vi "HFRR ADV v13.vi"() -> ()   [LabVIEW 2025] (continued)
                      n3139 = Fract/Exp String To Number(string=w4398) -> (number=→"Temperature before test 2":dbl)  [unwired: 3 in, 1 out]
                    }
                    frame 8 {
                      n3140 = Fract/Exp String To Number(string=w4400) -> (number=→"Humidity after test 2":dbl)  [unwired: 3 in, 1 out]
                    }
                    frame 9 {
                      n3141 = Fract/Exp String To Number(string=w4402) -> (number=→"Temperature after test 2":dbl)  [unwired: 3 in, 1 out]
                    }
                    frame 10 {
                      n3142 = Fract/Exp String To Number(string=w4404) -> (number=→"MWSD 2":dbl)  [unwired: 3 in, 1 out]
                    }
                    frame 11 {
                      n3143 = Fract/Exp String To Number(string=w4406) -> (number=→"AVP 2":dbl)  [unwired: 3 in, 1 out]
                    }
                    frame 12 {
                      n3144 = Fract/Exp String To Number(string=w4408) -> (number=→"HCF 2":dbl)  [unwired: 3 in, 1 out]
                    }
                    frame 13 {
                      n3145 = Fract/Exp String To Number(string=w4410) -> (number=→"WS1.4 2":dbl)  [unwired: 3 in, 1 out]
                    }
                    frame 14, Default {
                    }
                  }
                }
              }
              frame #2 {
              }
            }
            n3146 = local write "OK Button 16"(FALSE ("OK Button 13")) -> ()
          }
        }
        n3147 = Index Array(array=w4054, index="Select Printer 3") -> (element=w4056:string)
        "Selected Printer" <- w4056
        n3148 = case shown="True" w4051 {
          frame False {
          }
          frame True {
            n3149 = flat-sequence {
              frame #0 {
              }
              frame #1 {
                n3150 = Wait (ms)(milliseconds to wait=u32 100) -> ()  [unwired: 1 out]
              }
              frame #2 {
                n3151 = local write "OK Button 16"(FALSE ("Print 3")) -> ()
              }
            }
          }
        }
        n3152 = case shown="True" "Print" {
          tunnel: w4056 -> [_ w4348]
          frame False {
          }
          frame True {
            (unwired) i16 6 ("width (-)")
            (unwired) "TESTED BY : "
            (unwired) "TESTED DATE :"
            (unwired) "SAMPLE ID : "
            (unwired) "SAMPLE DESIGN : "
            w4306 = "\r"
            w4323 = "\r"
            # "add image"
            n3153 = local read "Sample ID"() -> (w4296:string)
            n3154 = local read "Tested by"() -> (w4299:string)
            n3155 = local read "String 34"() -> (w4286:string)
            n3156 = local read "String 45"() -> (w4266:string)
            n3157 = local read "String 35"() -> (w4281:string)
            n3158 = local read "String 37"() -> (w4279:string)
            n3159 = local read "String 32"() -> (w4301:string)
            n3160 = local read "String 36"() -> (w4276:string)
            n3161 = local read "String 31"() -> (w4300:string)
            n3162 = local read "Test Date"() -> (w4297:string)
            n3163 = local read "String 33"() -> (w4302:string)
            n3164 = local read "String 38"() -> (w4272:string)
            n3165 = local read "String 39"() -> (w4269:string)
            n3166 = local write "Print"(FALSE ("Print FF")) -> ()
            n3167 = local read "S 39"() -> (w4284:string)
            n3168 = local read "S 38"() -> (w4291:string)
            n3169 = local read "Temperature before test 2"() -> (w4322:dbl)
            n3170 = local read "Temperature after test 2"() -> (w4312:dbl)
            n3171 = local read "Humidity before test 2"() -> (w4337:dbl)
            n3172 = local read "Humidity after test 2"() -> (w4321:dbl)
            n3173 = local read "MWSD 2"() -> (w4326:dbl)
            n3174 = local read "WS1.4 2"() -> (w4304:dbl)
            n3175 = Concatenate Strings("2)" ("string"), w4286) -> (w4287:string)
            n3176 = Concatenate Strings("3)" ("string"), w4284) -> (w4285:string)
            n3177 = Concatenate Strings("1)" ("string"), w4291) -> (w4290:string)
            n3178 = Concatenate Strings("4)" ("string"), w4281) -> (w4282:string)
            n3179 = Concatenate Strings("5)" ("string"), w4279) -> (w4278:string)
            n3180 = Concatenate Strings("6)" ("string"), w4276) -> (w4275:string)
            n3181 = Concatenate Strings("7)" ("string"), w4272) -> (w4273:string)
            n3182 = Concatenate Strings("8)" ("string"), w4269) -> (w4270:string)
            n3183 = local read "HCF 2"() -> (w4308:dbl)
            n3184 = local read "AVP 2"() -> (w4325:dbl)
            n3185 = local read "s.NO"() -> (w4267:string)
            n3186 = call <vilib>:"New Report.vi"("report type"=enum16{"Standard Report", "HTML"}."Standard Report") -> ("report out"=w4346:refnum<class "NI_report.lvclass">, "error out"=w4345:errorcluster)  [unwired: 13 in]
            n3187 = local read "TITTLE"() -> (w4298:string)
            n3188 = Concatenate Strings(w4323, w4266, w4267, w4323, w4301, w4296, w4323, w4300, w4297, w4323, w4302, w4299, w4323) -> (w4316:string)
            "test by" <- w4316
            n3189 = Number To Fractional String(number=w4322, width (-)=i16 6, precision (6)=i16 2) -> (F-format string=w4311:string)  [unwired: 1 in]
            n3190 = Number To Fractional String(number=w4321, width (-)=i16 6, precision (6)=i16 2) -> (F-format string=w4324:string)  [unwired: 1 in]
            n3191 = Number To Fractional String(number=w4337, width (-)=i16 6, precision (6)=i16 2) -> (F-format string=w4342:string)  [unwired: 1 in]
            n3192 = Number To Fractional String(number=w4326, width (-)=i16 6, precision (6)=i16 2) -> (F-format string=w4328:string)  [unwired: 1 in]
            n3193 = Number To Fractional String(number=w4312, width (-)=i16 6, precision (6)=i16 2) -> (F-format string=w4313:string)  [unwired: 1 in]
            n3194 = Number To Fractional String(number=w4325, width (-)=i16 6, precision (6)=i16 2) -> (F-format string=w4327:string)  [unwired: 1 in]
            n3195 = Number To Fractional String(number=w4308, width (-)=i16 6, precision (6)=i16 2) -> (F-format string=w4307:string)  [unwired: 1 in]
            n3196 = Number To Fractional String(number=w4304, precision (6)=i16 2) -> (F-format string=w4303:string)  [unwired: 2 in]
            n3197 = call-dynamic "Set Report Header Text.vi"("report in"=w4346, "center header text"=w4298, "error in (no error)"=w4345) -> ("report out"=w4317:refnum<class "NI_report.lvclass">, "error out"=w4318:errorcluster)  [unwired: 11 in]
            n3198 = Concatenate Strings(w4306, w4290, w4342, w4306, w4287, w4311, w4306, w4285, w4324, w4306, w4282, w4313, w4306, w4278, w4328, w4306, w4275, w4327, w4306, w4273, w4307, w4306, w4270, w4303) -> (w4294:string)
            "export 2" <- w4294
            n3199 = call-poly <vilib>:"Append Report Text.vi"("report in"=w4317, "text"=w4316, "error in (no error)"=w4318) -> ("report out"=w4320:refnum<class "NI_report.lvclass">, "error out"=w4319:errorcluster)  [unwired: 9 in, 2 out]
            n3200 = local read "test by"() -> (w4293:string)
            n3201 = local read "TITTLE"() -> (w4295:string)
            n3202 = call-poly <vilib>:"Append Report Text.vi"("report in"=w4320, "error in (no error)"=w4319) -> ("report out"=w4341:refnum<class "NI_report.lvclass">, "error out"=w4339:errorcluster)  [unwired: 10 in, 2 out]
            n3203 = Concatenate Strings(w4295, w4294, w4293) -> (→"output":string)
            n3204 = call-poly <vilib>:"Append Report Text.vi"("report in"=w4341, "text"=w4294, "error in (no error)"=w4339) -> ("report out"=w4340:refnum<class "NI_report.lvclass">, "error out"=w4338:errorcluster)  [unwired: 9 in, 2 out]
            n3205 = call-dynamic "Print Report.vi"("report in"=w4340, "printer name (default)"=w4348, "error in (no error)"=w4338) -> ("report out"=w4350:refnum<class "NI_report.lvclass">, "error out"=w4351:errorcluster)  [unwired: 11 in]
            n3206 = call-dynamic "Dispose Report.vi"("report in"=w4350, "error in (no error)"=w4351) -> ()  [unwired: 13 in, 1 out]
          }
        }
        n3207 = case shown="True" "Print 2" {
          frame False {
          }
          frame True {
            n3208 = flat-sequence {
              frame #0 {
                n3209 = local read "s.NO"() -> (→"s.NO 2":string)
                n3210 = Wait (ms)(milliseconds to wait=u32 20) -> ()  [unwired: 1 out]
                n3211 = local read "Sample ID  3"() -> (→"Sample ID  6":string)
                n3212 = local read "Sample ID  4"() -> (→"Sample ID  7":string)
                n3213 = local read "Sample ID"() -> (→"Sample ID  2":string)
                n3214 = local read "Tested by"() -> (→"Tested by 2":string)
                n3215 = local read "Test Date"() -> (→"Test Date 2":string)
                n3216 = local read "Humidity after test 3"() -> (→"Humidity after test 4":dbl)
                n3217 = local read "Ref A Test Date :"() -> (→"TITTLE 4":string)
                n3218 = local read "Temperature before test 3"() -> (w4173:dbl)
                n3219 = local read "Temperature before test 3"() -> (→"Temperature after test 5":dbl)
                n3220 = local read "Temperature after test 3"() -> (→"Temperature after test 4":dbl)
                n3221 = local read "Humidity before test 3"() -> (→"Humidity before test 4":dbl)
                n3222 = local write "Temperature before test 3"(w4173) -> ()
                n3223 = local read "image data"() -> (w4164:T14)
                n3224 = String To Path(string="C:\\LAB-IQ\\im\\Temp_resized.jpg") -> (path=w4165:path)
                "path 2" <- w4165
                n3225 = call <vilib>:"Write JPEG File.vi"("image data"=w4164, "path to JPEG file"=w4165) -> ()  [unwired: 8 in, 2 out]
                "Ref A Test Date :" <- "Ref A Test Date :"
                "Ref B Test Date :" <- "Ref B Test Date :"
                "Ref B Scar Value :" <- "Ref B Scar Value :"
                "Ref A Scar Value :" <- "Ref A Scar Value :"
              }
              frame #1 {
                (unwired) HTML_Report_Image_Alignment."MIDDLE" ("alignment (default)")
                w4201 = u16 0 items=["portrait", "landscape"] ("orientation (portrait)")
                (unwired) HTML_Report_Image_Alignment."ABSMIDDLE" ("alignment (default)")
                (unwired) "TESTED BY : "
                (unwired) "TESTED DATE :"
                (unwired) "SAMPLE ID : "
                (unwired) "SAMPLE DESIGN : "
                w4234 = "\r"
                # "add image"
                n3226 = Wait (ms)(milliseconds to wait=u32 20) -> ()  [unwired: 1 out]
                n3227 = local read "Sample ID  2"() -> (w4227:string)
                n3228 = local read "Wear Scar X"() -> (w4199:dbl)
                "Length ( microns ) 2" <- w4199
                n3229 = local read "Wear Scar Y"() -> (w4198:dbl)
                "Wear Scar Y ( microns ) :" <- w4198
                n3230 = local read "Test Date 2"() -> (w4228:string)
                n3231 = local read "Tested by 2"() -> (w4229:string)
                n3232 = local read "String 46"() -> (w4225:string)
                n3233 = local read "String 48"() -> (w4231:string)
                n3234 = local read "String 47"() -> (w4230:string)
                n3235 = local read "String 49"() -> (w4232:string)
                n3236 = local read "String 10"() -> (w4185:string)
                n3237 = local read "s.NO 2"() -> (w4226:string)
                n3238 = Add(x=w4199, y=w4198) -> (x+y=w4197:dbl)
                n3239 = call <vilib>:"New Report.vi"("report type"=enum16{"Standard Report", "HTML"}."HTML") -> ("report out"=w4205:refnum<class "NI_report.lvclass">, "error out"=w4203:errorcluster)  [unwired: 13 in]
                n3240 = Concatenate Strings(w4234, w4225, w4226, w4234, w4231, w4227, w4234, w4230, w4228, w4234, w4232, w4229, w4234) -> (→"test by 2":string)
                n3241 = Concatenate Strings("C:\\LAB-IQ\\Data\\" ("string"), w4185, ".jpg" ("string")) -> ()  [unwired: 1 out]
                n3242 = Divide(x=w4197, y=2.0) -> (x/y=→"Mean Wear ( microns) :":dbl)
                n3243 = call-dynamic "Set Report Orientation.vi"("report in"=w4205, "orientation (portrait)"=w4201, "error in (no error)"=w4203) -> ("report out"=w4204:refnum<class "NI_report.lvclass">, "error out"=w4202:errorcluster)  [unwired: 11 in]
                n3244 = for {
                  N: 5 -> [_]
                  tunnel: w4204 -> [w4255]
                  tunnel: [w4254] -> w4183
                  tunnel: w4202 -> [w4253]
                  tunnel: [w4252] -> w4182
                  n3245 = call-dynamic "Set Report Tab Width.vi"("report in"=w4255, "error in (no error)"=w4253) -> ("report out"=w4254:refnum<class "NI_report.lvclass">, "error out"=w4252:errorcluster)  [unwired: 12 in]
                }
                n3246 = local read "TITTLE"() -> (w4200:string)
                n3247 = call-dynamic "Set Report Header Text.vi"("report in"=w4183, "center header text"=w4200, "error in (no error)"=w4182) -> ("report out"=w4221:refnum<class "NI_report.lvclass">, "error out"=w4220:errorcluster)  [unwired: 11 in]
                n3248 = for {
                  N: 1 -> [_]
                  tunnel: [w4259] -> w4207
                  tunnel: [w4258] -> w4206
                  tunnel: w4221 -> [w4257]
                  tunnel: w4220 -> [w4256]
                  n3249 = call-dynamic "New Report Line.vi"("report in"=w4257, "error in (no error)"=w4256) -> ("report out"=w4259:refnum<class "NI_report.lvclass">, "error out"=w4258:errorcluster)  [unwired: 12 in]
                }
                n3250 = for {
                  N: 2 -> [_]
                  tunnel: [w4251] -> w4213
                  tunnel: [w4250] -> w4212
                  tunnel: w4207 -> [w4249]
                  tunnel: w4206 -> [w4248]
                  n3251 = call-dynamic "New Report Line.vi"("report in"=w4249, "error in (no error)"=w4248) -> ("report out"=w4251:refnum<class "NI_report.lvclass">, "error out"=w4250:errorcluster)  [unwired: 12 in]
                }
                n3252 = for {
                  N: 25 -> [_]
                  tunnel: w4213 -> [w4247]
                  tunnel: w4212 -> [w4245]
                  tunnel: [w4246] -> w4216
                  tunnel: [w4244] -> w4215
                  n3253 = call-dynamic "Set Report Tab Width.vi"("report in"=w4247, "error in (no error)"=w4245) -> ("report out"=w4246:refnum<class "NI_report.lvclass">, "error out"=w4244:errorcluster)  [unwired: 12 in]
                }
                n3254 = control-ref of="Tab Control 9"() -> (w4211:refnum<vi>)
                n3255 = call-dynamic "Append Control Image to Report.vi"("report in"=w4216, "alignment (default)"=HTML_Report_Image_Alignment."ABSMIDDLE", "ctrl reference"=w4211, "error in (no error)"=w4215) -> ("report out"=w4210:refnum<class "NI_report.lvclass">, "error out"=w4209:errorcluster)  [unwired: 8 in, 2 out]
                n3256 = for {
                  N: 3 -> [_]
                  tunnel: [w4243] -> w4194
                  tunnel: [w4242] -> w4193
                  tunnel: w4210 -> [w4241]
                  tunnel: w4209 -> [w4240]
                  n3257 = call-dynamic "New Report Line.vi"("report in"=w4241, "error in (no error)"=w4240) -> ("report out"=w4243:refnum<class "NI_report.lvclass">, "error out"=w4242:errorcluster)  [unwired: 12 in]
                }
                n3258 = for {
                  N: 100 -> [_]
                  tunnel: w4194 -> [w4239]
                  tunnel: w4193 -> [w4237]
                  tunnel: [w4238] -> w4190
                  tunnel: [w4236] -> w4188
                  n3259 = call-dynamic "Set Report Tab Width.vi"("report in"=w4239, "error in (no error)"=w4237) -> ("report out"=w4238:refnum<class "NI_report.lvclass">, "error out"=w4236:errorcluster)  [unwired: 12 in]
                }
                n3260 = String To Path(string="C:\\LAB-IQ\\im\\Temp_resized.jpg") -> (path=w4180:path)
                n3261 = call-poly <vilib>:"Append Image to Report.vi"("report in"=w4190, "path or URL of image"=w4180, "error in (no error)"=w4188) -> ("report out"=w4189:refnum<class "NI_report.lvclass">, "error out"=w4187:errorcluster)  [unwired: 9 in, 2 out]
                n3262 = call-poly <vilib>:"Open HTML Report in Browser.vi"("report in"=w4189, "error in (no error)"=w4187) -> ("report out"=w4224:refnum<class "NI_report.lvclass">, "error out"=w4223:errorcluster)  [unwired: 11 in, 1 out]
                n3263 = call-dynamic "Dispose Report.vi"("report in"=w4224, "error in (no error)"=w4223) -> ()  [unwired: 13 in, 1 out]
              }
              frame #2 {
              }
              frame #3 {
                n3264 = disable-structure shown="Disabled" {
                  frame Disabled {
                    n3265 = local read "String 10"() -> (w4264:string)
                    n3266 = Concatenate Strings("C:\\LAB-IQ-NXT\\Data\\" ("string"), w4264, ".jpg" ("string")) -> (w4262:string)
                    n3267 = String To Path(string=w4262) -> (path=w4261:path)
                    n3268 = Delete(path (use dialog)=w4261) -> ()  [unwired: 4 in, 3 out]
                  }
                  frame Enabled {
                  }
                }
                n3269 = local write "Print 2"(FALSE ("Print")) -> ()
              }
            }
          }
        }
      }
    }
    n3270 = property on="SetTemp" class="DigNum (strict)"("Disabled"=w2148) -> ()  [unwired: 2 in, 2 out]
    n3271 = Multiply(x=w2137, y=w2139) -> (x*y=w2138:dbl)
    n3272 = local read "MWSD"() -> (w2136:dbl)
    n3273 = Add(x=w2138, y=w2136) -> (x+y=→"WS1.4":dbl)
    n3274 = Wait (ms)(milliseconds to wait=u32 50) -> ()  [unwired: 1 out]
    n3275 = Wait (ms)(milliseconds to wait=u32 50) -> ()  [unwired: 1 out]
    n3276 = local read "Quit"() -> (w2135:bool)
  }
  n3277 = VISA Close(VISA resource name=w53, error in (no error)=w52) -> (error out=w50:errorcluster)
  n3278 = VISA Close(VISA resource name=w34, error in (no error)=w33) -> ()  [unwired: 1 out]
  n3279 = call <vilib>:"Clear Errors.vi"("error in (no error)"=w50) -> ()  [unwired: 5 in, 2 out]
  n3280 = Or(x=w40, y=w39) -> (x .or. y?=w41:bool)
  n3281 = while {
    tunnel: [w4412] -> w46
    shift-right: [w4450] -> _
    shift-left: "" -> [w4438]
    tunnel: [w4426] -> _
    i -> [w4426]
    stop <- w4412 stop-if-true
    w4452 = ";" ("string")
    n3282 = local read "start en"() -> (w4471:bool)
    n3283 = And(x="st enable", y=w4471) -> (x .and. y?=w4472:bool)
    n3284 = local read "Elapsed time"() -> (w4434:dbl)
    n3285 = local read "ACQUIRE 3"() -> (w4415:bool)
    n3286 = case shown="True" w4472 {
      tunnel: "st enable" -> [w4536 w4537]
      tunnel: [w4536 w4537] -> w4416
      frame False {
      }
      frame True {
        n3287 = local write "start en"(FALSE ("start en")) -> ()
      }
    }
    n3288 = Wait (ms)(milliseconds to wait=u32 80) -> ()  [unwired: 1 out]
    n3289 = local read "Stroke"() -> (w4425:dbl)
    n3290 = Greater?(x=w4434, y=0.1) -> (0:w4432:bool)
    n3291 = Or(x=w4416, y=w4415) -> (x .or. y?=w4417:bool)
    n3292 = case shown="True" "ACQUIRE 2" {
      frame False {
      }
      frame True {
        n3293 = call "Elapsed Time13"() -> ("Time has Elapsed"=w4479:bool)  [unwired: 12 in, 7 out]
        n3294 = case shown="True" w4479 {
          frame False {
          }
          frame True {
            n3295 = local write "ACQUIRE 2"(FALSE ("ACQUIRE 2")) -> ()
            n3296 = local write "ACQUIRE 3"(FALSE ("ACQUIRE 2")) -> ()
          }
        }
        n3297 = local write "ACQUIRE 3"(TRUE ("ACQUIRE 2")) -> ()
      }
    }
    n3298 = case shown="True" w4417 {
      tunnel: w4425 -> [_ w4559]
      tunnel: [w4539 _] -> w4469
      tunnel: w4432 -> [_ _]
      tunnel: w4415 -> [_ w4546]
      frame False {
        w4539 = TRUE ("PID Rst")
        n3299 = local read "stop cmd"() -> (w4540:bool)
        n3300 = case shown="True" w4540 {
          frame False {
          }
          frame True {
            n3301 = local write "stop cmd"(FALSE ("stop cmd")) -> ()
          }
        }
        n3302 = local write "PID Rst"(TRUE ("PID Rst")) -> ()
        "start en" <- w4539
      }
      frame True {
        w4566 = cluster{"output high":dbl, "output low":dbl} {"output high"=600.0, "output low"=-600.0} ("output range")
        n3303 = local read "STROKE GAIN :"() -> (w4551:dbl)
        n3304 = call "Elapsed Time6"("Reset"="PID Rst", "Auto Reset"=FALSE) -> ("Time has Elapsed"=w4560:bool)  [unwired: 10 in, 7 out]
        n3305 = Multiply(x="Set Strk", y=w4551) -> (x*y=w4544:dbl)
        n3306 = case shown="False" w4560 {
          tunnel: [w4571 w4572] -> w4563
          tunnel: "Set Strk" -> [w4571 _]
          tunnel: w4559 -> [_ w4572]
          frame False {
          }
          frame True {
          }
        }
        n3307 = Multiply(x=w4544, y=1.0) -> (x*y=w4543:dbl)
        n3308 = Select(t=T9 {"Proportional Gain (Kc)"=0.0, "Integral Time (Ti, min)"=0.02, "Derivative Time (Td, min)"=0.0} ("Stroke PID Gains"), s=w4546, f="Stroke PID Gains") -> (s? t:f=w4547:T9)
        n3309 = Not(x=w4560) -> (.not. x?=w4558:bool)
        n3310 = call-poly <vilib>:"PID.vi"("reinitialize? (F)"=w4558, "output range"=w4566, "PID gains"=w4547, "process variable"=w4563, "setpoint"="Set Strk") -> ("output"=w4557:dbl)  [unwired: 5 in, 1 out]
        "Stroke PID OUT" <- w4557
        n3311 = Select(t=w4557, s=w4560, f=0.0) -> (s? t:f=w4561:dbl)
        n3312 = flat-sequence {
          tunnel: w4561 -> [_]
          frame #0 {
            n3313 = local write "PID Rst"(FALSE ("PID Rst")) -> ()
          }
        }
        n3314 = Add(x=w4543, y=w4561) -> (x+y=w4556:dbl)
        n3315 = Unbundle(w4566) -> ("output high"=w4565:dbl, "output low"=w4564:dbl)
        n3316 = To Word Integer(number=w4556) -> (16bit integer=w4553:i16)
        n3317 = property on="Stroke PID OUT" class="Slide (strict)"("Scale.Range:Minimum"=w4564, "Scale.Range:Maximum"=w4565) -> ()  [unwired: 2 in, 2 out]
        n3318 = In Range and Coerce(upper limit=4095.0 ("f"), x=w4553, lower limit=100.0 ("f")) -> (coerced(x)=w4550:dbl)  [unwired: 1 out]
        "PID Out" <- w4550
        n3319 = Number To Decimal String(number=w4550) -> (decimal integer string=→"st gain":string)  [unwired: 1 in]
        "stop cmd" <- TRUE ("Auto Reset")
      }
    }
    n3320 = flat-sequence {
      frame #0 {
        n3321 = local read "CH-POWER +"() -> (w4483:u16)
        n3322 = local read "CH-POWER -"() -> (w4484:u16)
        n3323 = case shown="1" w4484 {
          tunnel: "PWR" -> [w4485 w4486 w4487 w4488 w4489 w4490 w4491 w4492]
          frame 0, Default {
            n3324 = local write "Do 0"(w4485) -> ()
          }
          frame 1 {
            n3325 = local write "Do 1"(w4486) -> ()
          }
          frame 2 {
            n3326 = local write "Do 2"(w4487) -> ()
          }
          frame 3 {
            n3327 = local write "Do 3"(w4488) -> ()
          }
          frame 4 {
            n3328 = local write "Do 4"(w4489) -> ()
          }
          frame 5 {
            n3329 = local write "Do 5"(w4490) -> ()
          }
          frame 6 {
            n3330 = local write "Do 6"(w4491) -> ()
          }
          frame 7 {
            n3331 = local write "Do 7"(w4492) -> ()
          }
        }
        n3332 = case shown="1" w4483 {
          tunnel: "PWR" -> [w4493 w4494 w4495 w4496 w4497 w4498 w4499 w4500]
          frame 0, Default {
            n3333 = local write "Do 0"(w4493) -> ()
          }
          frame 1 {
            n3334 = local write "Do 1"(w4494) -> ()
          }
          frame 2 {
            n3335 = local write "Do 2"(w4495) -> ()
          }
          frame 3 {
            n3336 = local write "Do 3"(w4496) -> ()
          }
          frame 4 {
            n3337 = local write "Do 4"(w4497) -> ()
          }
          frame 5 {
            n3338 = local write "Do 5"(w4498) -> ()
          }
          frame 6 {
            n3339 = local write "Do 6"(w4499) -> ()
          }
          frame 7 {
            n3340 = local write "Do 7"(w4500) -> ()
          }
        }
      }
    }
    n3341 = local read "RUN"() -> (w4423:bool)
    n3342 = Or(x=w4423, y="ACQUIRE 3") -> (x .or. y?=w4422:bool)
    n3343 = local read "Set Hz"() -> (w4440:dbl)
    n3344 = Select(t=w4440, s=w4422, f=0.0) -> (s? t:f=w4439:dbl)
    n3345 = local read "st gain"() -> (w4443:string)
    n3346 = local read "DO"() -> (w4444:string)
    n3347 = case shown="True" "Boolean 10" {
      frame False {
      }
      frame True {
        n3348 = local write "Tab Control 8"(enum32{"setup", "calibrate"}."calibrate" ("Tab Control 8")) -> ()
        n3349 = local write "Boolean 10"(FALSE ("Boolean 10")) -> ()
      }
    }
    n3350 = Number To Decimal String(number=w4439) -> (decimal integer string=w4442:string)  [unwired: 1 in]
    n3351 = case shown="True" "Boolean 11" {
      frame False {
      }
      frame True {
        n3352 = local write "Tab Control 8"(enum32{"setup", "calibrate"}."setup" ("Tab Control 8")) -> ()
        n3353 = local write "Boolean 11"(FALSE ("Boolean 11")) -> ()
      }
    }
    n3354 = String Length(string=w4443) -> (length=w4458:i32)
    n3355 = String Length(string=w4444) -> (length=w4446:i32)
    n3356 = String Length(string=w4442) -> (length=w4459:i32)
    n3357 = Subtract(x=4.0, y=w4458) -> (x-y=w4455:dbl)
    n3358 = Subtract(x=3.0, y=w4446) -> (x-y=w4449:dbl)
    n3359 = flat-sequence {
      tunnel: w4469 -> [_]
      frame #0 {
        n3360 = Build Array("Do 0", "Do 1", "Do 2", "Do 3", "Do 4", "Do 5", "Do 6", "Do 7") -> (w4527:bool[])
        n3361 = Boolean Array To Number(Boolean array=w4527) -> (number=w4525:u32)
        n3362 = Add(x=w4525, y=u32 0) -> (x+y=w4523:u32)
        n3363 = Number To Decimal String(number=w4523) -> (decimal integer string=→"DO":string)  [unwired: 1 in]
      }
    }
    n3364 = Subtract(x=3.0, y=w4459) -> (x-y=w4460:dbl)
    n3365 = Replace Substring(3:w4455, 4:w4443, 5:"0000" ("string")) -> (1:w4453:string)  [unwired: 1 in, 1 out]
    n3366 = Replace Substring(3:w4449, 4:w4444, 5:"000" ("string")) -> (1:w4445:string)  [unwired: 1 in, 1 out]
    n3367 = Replace Substring(3:w4460, 4:w4442, 5:"000" ("string")) -> (1:w4454:string)  [unwired: 1 in, 1 out]
    n3368 = Concatenate Strings("*" ("string"), w4454, w4452, w4453, w4452, w4445, "$" ("string")) -> (w4450:string)
    "Stroke_send_Val" <- w4450
    n3369 = local read "RUN"() -> (w4420:bool)
    n3370 = local read "ACQUIRE 3"() -> (w4419:bool)
    n3371 = local read "send"() -> (w4436:bool)
    n3372 = Not Equal?(x=w4438, y=w4450) -> (x != y?=w4451:bool)
    n3373 = Or(x=w4420, y=w4419) -> (x .or. y?=w4418:bool)
    n3374 = And(x=w4436, y=w4418) -> (x .and. y?=w4435:bool)
    n3375 = Or(x=w4451, y=w4435) -> (x .or. y?=w4429:bool)
    n3376 = case shown="False" w4418 {
      frame False {
        "send" <- TRUE ("send")
      }
      frame True {
      }
    }
    n3377 = call "Elapsed Time4"("Time Target (s)"=0.5) -> ("Time has Elapsed"=w4427:bool)  [unwired: 11 in, 7 out]
    n3378 = local read "Din"() -> (w4468:u8[])
    n3379 = Or(x=w4427, y=w4429) -> (x .or. y?=w4428:bool)
    n3380 = local read "Quit"() -> (w4412:bool)
    n3381 = Index Array(array=w4468, index=0) -> (element=w4466:u8)
    n3382 = case shown="True" w4428 {
      tunnel: w4450 -> [_ w4504]
      frame False {
      }
      frame True {
        n3383 = local read "Due Com"() -> (w4505:string[])
        n3384 = Build Array (concatenate)(w4505, w4504) -> (→"Due Com":string[])
        n3385 = local write "send"(FALSE ("send")) -> ()
      }
    }
    n3386 = Number To Boolean Array(number=w4466) -> (Boolean array=w4465:bool[])
    n3387 = Array Size(array=w4465) -> (size(s)=w4464:i32)
    n3388 = Greater Than 0?(x=w4464) -> (x > 0?=w4463:bool)
    n3389 = case shown="True" w4463 {
      tunnel: w4465 -> [_ w4519]
      frame False {
      }
      frame True {
        n3390 = Index Array(array=w4519, index #1=0 ("index"), index #2=1 ("index"), index #3=2 ("index"), index #4=3 ("index"), index #5=4 ("index"), index #6=5 ("index"), index #7=6 ("index"), index #8=7 ("index")) -> (element #1=→"DI 0":bool, element #2=→"DI 1":bool, element #3=→"DI 2":bool, element #4=→"DI 3":bool, element #5=→"DI 4":bool, element #6=→"DI 5":bool, element #7=→"DI 6":bool, element #8=→"DI 7":bool)
      }
    }
  }
  n3391 = Or(x=w36, y=w41) -> (x .or. y?=w48:bool)
  n3392 = control-ref of="new picture"() -> ()  [unwired: 1 out]
  n3393 = Or(x=w55, y=w48) -> (x .or. y?=w45:bool)
  n3394 = Or(x=w45, y=w46) -> (x .or. y?=w37:bool)
  n3395 = while {
    tunnel: [w4574] -> w59
    tunnel: [w4575] -> _
    i -> [w4575]
    stop <- w4574 stop-if-true
    n3396 = local read "PID-out"() -> (w4576:dbl)
    "Horizontal Slider Control" <- w4576
    n3397 = Greater Or Equal?(x=w4576, y=2.0) -> (x >= y?=w4577:bool)
    n3398 = flat-sequence {
      tunnel: w4577 -> [w4585]
      tunnel: w4576 -> [w4588]
      tunnel: [w4586] -> w4583
      tunnel: [w4584] -> w4582
      tunnel: [w4604] -> w4581
      tunnel: w4583 -> [w4604]
      tunnel: w4582 -> [w4601]
      tunnel: [w4601] -> w4580
      tunnel: w4581 -> [w4606]
      tunnel: [w4605] -> w4579
      tunnel: w4580 -> [w4605]
      tunnel: w4579 -> [w4620]
      frame #0 {
        n3399 = case shown="True" w4585 {
          selector: w4585 -> [w4590 _]
          frame False {
            n3400 = local write "HEATER"(w4590) -> ()
          }
          frame True {
            w4592 = TRUE ("data")
            n3401 = local read "CH-HEATER"() -> (w4591:u16)
            n3402 = case shown="2" w4591 {
              tunnel: w4592 -> [w4593 w4594 w4595 w4596 w4597 w4598 w4599 w4600]
              frame 0, Default {
                n3403 = local write "Do 0"(w4593) -> ()
              }
              frame 1 {
                n3404 = local write "Do 1"(w4594) -> ()
              }
              frame 2 {
                n3405 = local write "Do 2"(w4595) -> ()
              }
              frame 3 {
                n3406 = local write "Do 3"(w4596) -> ()
              }
              frame 4 {
                n3407 = local write "Do 4"(w4597) -> ()
              }
              frame 5 {
                n3408 = local write "Do 5"(w4598) -> ()
              }
              frame 6 {
                n3409 = local write "Do 6"(w4599) -> ()
              }
              frame 7 {
                n3410 = local write "Do 7"(w4600) -> ()
              }
            }
            "HEATER" <- w4592
          }
        }
        n3411 = Select(t=w4588, s=w4585, f=0.0) -> (s? t:f=w4584:dbl)
        n3412 = Greater Or Equal?(x=w4588, y=97.0) -> (x >= y?=w4586:bool)
      }
      frame #1 {
        n3413 = Multiply(x=w4601, y=5.0) -> (x*y=w4603:dbl)
        n3414 = Wait (ms)(milliseconds to wait=w4603) -> ()  [unwired: 1 out]
      }
      frame #2 {
        n3415 = case shown="False" w4606 {
          frame False {
            w4607 = FALSE ("data")
            n3416 = local read "CH-HEATER"() -> (w4608:u16)
            n3417 = case shown="4" w4608 {
              tunnel: w4607 -> [w4609 w4610 w4611 w4612 w4613 w4614 w4615 w4616]
              frame 0, Default {
                n3418 = local write "Do 0"(w4609) -> ()
              }
              frame 1 {
                n3419 = local write "Do 1"(w4610) -> ()
              }
              frame 2 {
                n3420 = local write "Do 2"(w4611) -> ()
              }
              frame 3 {
                n3421 = local write "Do 3"(w4612) -> ()
              }
              frame 4 {
                n3422 = local write "Do 4"(w4613) -> ()
              }
              frame 5 {
                n3423 = local write "Do 5"(w4614) -> ()
              }
              frame 6 {
                n3424 = local write "Do 6"(w4615) -> ()
              }
              frame 7 {
                n3425 = local write "Do 7"(w4616) -> ()
              }
            }
            n3426 = local write "HEATER"(w4607) -> ()
          }
          frame True {
          }
        }
      }
      frame #3 {
        n3427 = Subtract(x=100, y=w4620) -> (x-y=w4619:dbl)
        n3428 = Multiply(x=w4619, y=5.0) -> (x*y=w4617:dbl)
        n3429 = Wait (ms)(milliseconds to wait=w4617) -> ()  [unwired: 1 out]
      }
    }
    n3430 = local read "Quit"() -> (w4574:bool)
  }
  n3431 = Or(x=w59, y=w37) -> (x .or. y?=w58:bool)
  n3432 = while {
    tunnel: [w4622] -> w54
    i -> [w4629]
    stop <- w4622 stop-if-true
    n3433 = local read "Quit"() -> (w4622:bool)
    n3434 = Equal To 0?(x=w4629) -> (x = 0?=w4627:bool)
    n3435 = call "Elapsed Time3"("Time Target (s)"=45.0, "Auto Reset"=TRUE) -> ("Time has Elapsed"=w4626:bool)  [unwired: 10 in, 7 out]
    n3436 = Wait (ms)(milliseconds to wait=u32 50) -> ()  [unwired: 1 out]
    n3437 = Or(x=w4626, y=w4627) -> (x .or. y?=w4628:bool)
    n3438 = case shown="True" w4628 {
      frame False {
      }
      frame True {
        n3439 = call <vilib>:"System Exec.vi"("run minimized? (F)"=TRUE, "error in (no error)"="error in (no error)", "command line"="powercfg.exe -change -monitor-timeout-ac 0") -> ("error out"=w4640:errorcluster)  [unwired: 5 in, 3 out]
        n3440 = call <vilib>:"System Exec.vi"("run minimized? (F)"=TRUE, "error in (no error)"=w4640, "command line"="powercfg.exe -change -disk-timeout-ac 0") -> ("error out"=w4639:errorcluster)  [unwired: 5 in, 3 out]
        n3441 = call <vilib>:"System Exec.vi"("run minimized? (F)"=TRUE, "error in (no error)"=w4639, "command line"="powercfg.exe -change -standby-timeout-ac 0") -> ("error out"=w4638:errorcluster)  [unwired: 5 in, 3 out]
        n3442 = call <vilib>:"System Exec.vi"("run minimized? (F)"=TRUE, "error in (no error)"=w4638, "command line"="powercfg.exe -change -hibernate-timeout-ac 0") -> ("error out"=w4637:errorcluster)  [unwired: 5 in, 3 out]
        n3443 = call <vilib>:"Simple Error Handler.vi"("error in (no error)"=w4637) -> ("error out"=w4643:errorcluster)  [unwired: 4 in, 4 out]
        n3444 = call <vilib>:"Clear Errors.vi"("error in (no error)"=w4643) -> ("error out"=→"error out":errorcluster)  [unwired: 5 in, 1 out]
      }
    }
  }
  n3445 = Compound Arithmetic op=OR(w57, w58, w54) -> (w56:bool)
  n3446 = flat-sequence {
    tunnel: w56 -> [_]
    tunnel: [w4645] -> w14
    tunnel: w14 -> [_]
    frame #0 {
      n3447 = call "CLOSE CONNECTION.vi"() -> ("error out"=w4645:errorcluster)  [unwired: 11 in]
    }
    frame #1 {
      n3448 = Quit LabVIEW(quit? (T)=TRUE) -> ()
      n3449 = local write "Quit"(FALSE ("EXIT")) -> ()
    }
  }
  n3450 = property on="Heater Button" class="Bool (strict)"("Visible"=TRUE) -> ()  [unwired: 2 in, 2 out]
  n3451 = disable-structure shown="Disabled" {
    disable-tunnel: _ -> [w4651 _]
    disable-tunnel: _ -> [w4648 _]
    disable-tunnel: _ -> [w4649 _]
    frame Disabled {
      n3452 = disable-structure shown="Disabled" {
        disable-tunnel: [w4658 _] -> w4650
        frame Disabled {
          n3453 = while {
            shift-right: [w4700] -> w4656
            shift-left: errorcluster {"status"=TRUE, "code"=0, "source"="Init"} ("error out") -> [w4665]
            shift-right: [w4699] -> w4655
            shift-left: _ -> [w4666]
            shift-right: [w4698] -> _
            shift-left: "" -> [w4697]
            tunnel: [w4659] -> w4658
            shift-right: ["Set Rh"] -> _
            shift-left: 0.0 ("Set Rh") -> [w4691]
            tunnel: [w4668] -> _
            i -> [w4668]
            stop <- w4659 stop-if-true
            n3454 = flat-sequence {
              tunnel: w4665 -> [w4703]
              tunnel: [w4703] -> w4664
              frame #0 {
                n3455 = Wait (ms)(milliseconds to wait=u32 200) -> ()  [unwired: 1 out]
              }
            }
            n3456 = local read "Com Port 3"() -> (w4667:refnum<visa-resource-name>)
            n3457 = local read "Humidity Str Rec"() -> (w4669:string)
            n3458 = Not Equal?(x="Set Rh", y=w4691) -> (x != y?=w4696:bool)
            n3459 = Number To Decimal String(number="Set Rh") -> (decimal integer string=w4694:string)  [unwired: 1 in]
            n3460 = Not Equal?(x=w4667, y=w4666) -> (x != y?=w4662:bool)
            n3461 = Concatenate Strings("#setPoint00" ("string"), w4694) -> (w4695:string)
            n3462 = case shown="False" w4696 {
              tunnel: w4695 -> [_ w4715]
              frame False {
                n3463 = local read "Humidity"() -> (w4712:bool)
                n3464 = case shown="True" w4712 {
                  frame False {
                    n3465 = local write "Humidity Str Send"("stop" ("Humidity Str Send")) -> ()
                  }
                  frame True {
                    n3466 = local write "Humidity Str Send"("start" ("Humidity Str Send")) -> ()
                  }
                }
              }
              frame True {
                n3467 = local write "Humidity Str Send"(w4715) -> ()
              }
            }
            n3468 = Or(x=w4662, y="Re-Initialise") -> (x .or. y?=w4661:bool)
            n3469 = String Subset(string=w4669, offset (0)=7) -> (substring=w4684:string)  [unwired: 1 in]
            n3470 = Match Pattern(string=w4669, regular expression="?") -> (offset past match=w4687:i32)  [unwired: 1 in, 3 out]
            n3471 = Match Pattern(string=w4669, regular expression="v") -> (offset past match=w4690:i32)  [unwired: 1 in, 3 out]
            n3472 = case shown="True" w4661 {
              tunnel: w4664 -> [w4701 _]
              tunnel: [w4701 errorcluster {"status"=TRUE, "code"=0, "source"="Init"} ("error out")] -> w4663
              frame False {
              }
              frame True {
              }
            }
            n3473 = Equal?(x=w4687, y=-1) -> (x = y?=w4671:bool)
            n3474 = Match Pattern(string=w4684, regular expression="g") -> (after substring=w4685:string, offset past match=w4676:i32)  [unwired: 1 in, 2 out]
            n3475 = Match Pattern(string=w4684, regular expression="y") -> (after substring=w4683:string, offset past match=w4677:i32)  [unwired: 1 in, 2 out]
            n3476 = Greater?(x=w4677, y=w4676) -> (0:w4682:bool)
            n3477 = Greater Or Equal To 0?(x=w4677) -> (x >= 0?=w4674:bool)
            n3478 = Greater Or Equal To 0?(x=w4676) -> (x >= 0?=w4675:bool)
            n3479 = Or(x=w4674, y=w4675) -> (x .or. y?=w4673:bool)
            n3480 = Greater Or Equal To 0?(x=w4690) -> (x >= 0?=w4672:bool)
            n3481 = Select(t=w4683, s=w4682, f=w4685) -> (s? t:f=w4678:string)
            n3482 = case shown="Error" w4663 {
              selector: w4663 -> [w4728 w4774]
              tunnel: [w4726 w4767] -> w4700
              tunnel: w4666 -> [w4729 w4773]
              tunnel: [w4727 w4776] -> w4699
              tunnel: w4697 -> [w4716 w4775]
              tunnel: [w4723 w4775] -> w4698
              frame No Error {
                n3483 = call "Elapsed Time7"() -> ("Time has Elapsed"=w4722:bool)  [unwired: 12 in, 7 out]
                n3484 = Not Equal?(x="Humidity Str Send", y=w4716) -> (x != y?=w4718:bool)
                n3485 = Or(x=w4718, y=w4722) -> (x .or. y?=w4721:bool)
                n3486 = Select(t="Humidity Str Send", s=w4718, f="vals" ("regular expression")) -> (s? t:f=w4717:string)
                n3487 = Or(x=w4721, y="Send") -> (x .or. y?=w4725:bool)
                n3488 = case shown="True" w4725 {
                  tunnel: [w4732 w4737] -> w4726
                  tunnel: w4729 -> [w4731 w4745]
                  tunnel: w4728 -> [w4732 w4744]
                  tunnel: [w4731 w4738] -> w4727
                  tunnel: w4717 -> [_ w4743]
                  tunnel: [w4730 w4734] -> w4723
                  tunnel: "Humidity Str Send" -> [_ w4735]
                  tunnel: w4718 -> [_ w4736]
                  tunnel: w4716 -> [w4730 w4733]
                  frame False {
                  }
                  frame True {
                    n3489 = flat-sequence {
                      tunnel: w4745 -> [w4753]
                      tunnel: w4744 -> [w4752]
                      tunnel: w4743 -> [w4749]
                      tunnel: [w4751] -> w4742
                      tunnel: [w4750] -> w4741
                      tunnel: w4742 -> [w4756]
                      tunnel: w4741 -> [w4755]
                      tunnel: [w4756] -> w4740
                      tunnel: [w4755] -> w4739
                      tunnel: w4740 -> [w4763]
                      tunnel: w4739 -> [w4762]
                      tunnel: [w4761] -> w4738
                      tunnel: [w4760] -> w4737
                      frame #0 {
                        n3490 = local write "Ser Led"(TRUE ("Boolean 4")) -> ()
                        n3491 = Concatenate Strings(w4749, "\r") -> (w4748:string)
                        n3492 = VISA Write(VISA resource name=w4753, write buffer=w4748, error in (no error)=w4752) -> (VISA resource name out=w4751:refnum<visa-resource-name>, error out=w4750:errorcluster)  [unwired: 1 out]
                      }
                      frame #1 {
                        n3493 = Wait (ms)(milliseconds to wait="wait") -> ()  [unwired: 1 out]
                      }
                      frame #2 {
                        w4758 = FALSE ("Send")
                        n3494 = property class="Instr"(reference=w4763, error in=w4762) -> (reference out=w4764:refnum<visa-resource-name>, error out=w4765:errorcluster, "Serial Settings:Number of Bytes at Serial Port"=w4757:u32)
                        "Humidity 2" <- w4757
                        n3495 = local write "Send"(w4758) -> ()
                        n3496 = local write "Ser Led"(w4758) -> ()
                        n3497 = VISA Read(VISA resource name=w4764, byte count=w4757, error in (no error)=w4765) -> (VISA resource name out=w4761:refnum<visa-resource-name>, read buffer=→"Humidity Str Rec":string, error out=w4760:errorcluster)  [unwired: 1 out]
                      }
                    }
                    n3498 = Select(t=w4735, s=w4736, f=w4733) -> (s? t:f=w4734:string)
                  }
                }
              }
              frame Error {
                w4781 = u16 0 items=["None"=0, "XON/XOFF"=1, "RTS/CTS"=2, "DTR/DSR"=4] ("flow control")
                w4777 = u16 0 items=["None", "Odd", "Even", "Mark", "Space"] ("parity")
                w4780 = u16 10 items=["1.0"=10, "1.5"=15, "2.0"=20] ("stop bits")
                n3499 = VISA Close(VISA resource name=w4773, error in (no error)=w4774) -> (error out=w4772:errorcluster)
                n3500 = local write "humid"("" ("humid")) -> ()
                n3501 = local write "Humidity Str Rec"("" ("Humidity Str Rec")) -> ()
                n3502 = call <vilib>:"Clear Errors.vi"("error in (no error)"=w4772) -> ("error out"=w4771:errorcluster)  [unwired: 5 in, 1 out]
                n3503 = local read "Com Port 3"() -> (w4770:refnum<visa-resource-name>)
                n3504 = call-poly "VISA Configure Serial Port"("VISA resource name"=w4770, "timeout (10sec)"=u32 1000, "termination char\n(0xA = '\\n' = LF)"=u8 10 ("termination char\n(0xA = '\\n' = LF)"), "Enable Termination\nChar (T)"=FALSE ("Enable Termination Char (T)"), "baud rate (9600)"="Humidity BaudRate", "data bits (8)"=u16 8 ("data bits"), "parity (0:none)"=w4777, "error in (no error)"=w4771, "stop bits (10: 1 bit)"=w4780, "flow control (0:none)"=w4781) -> ("VISA resource name out"=w4776:refnum<visa-resource-name>, "error out"=w4767:errorcluster)  [unwired: 4 in]
              }
            }
            n3505 = Compound Arithmetic op=AND(w4672, w4671, w4673) -> (w4670:bool)
            n3506 = case shown="True" w4670 {
              tunnel: w4669 -> [_ _]
              tunnel: w4678 -> [_ w4708]
              frame False {
              }
              frame True {
                w4706 = " " ("regular expression")
                n3507 = Match Pattern(string=w4708, regular expression=" ") -> (after substring=w4710:string)  [unwired: 1 in, 3 out]
                n3508 = Match Pattern(string=w4710, regular expression=w4706) -> (before substring=→"humid":string, after substring=w4707:string)  [unwired: 1 in, 2 out]
                n3509 = Match Pattern(string=w4707, regular expression=w4706) -> (before substring=→"temp_@Rh sensor":string)  [unwired: 1 in, 3 out]
              }
            }
            n3510 = local read "Quit"() -> (w4659:bool)
          }
          n3511 = VISA Close(VISA resource name=w4655, error in (no error)=w4656) -> (error out=w4652:errorcluster)
          n3512 = call <vilib>:"Clear Errors.vi"("error in (no error)"=w4652) -> ()  [unwired: 5 in, 2 out]
        }
        frame Enabled {
        }
      }
    }
    frame Enabled {
    }
  }
  n3513 = while {
    tunnel: [w4789] -> _
    i -> [w4789]
    stop <- w4784 stop-if-true
    # "Langauage selection"
    n3514 = property on="FF Calibration g" class="WFGraph (strict)"("Plot Area:Colors:FG Color"=u32 0) -> ()  [unwired: 2 in, 2 out]
    n3515 = Equal?(x="Lan flag", y=22.0) -> ()  [unwired: 1 out]
    n3516 = disable-structure shown="Disabled" {
      frame Disabled {
        n3517 = stacked-sequence {
          frame #0 {
            n3518 = case shown="\"Russian\"" "Language Selection" {
              tunnel: [0 1] -> w4791
              frame "English", Default {
              }
              frame "Russian" {
              }
            }
            n3519 = for {
              N: 130 -> [_]
              tunnel: "Table" -> [w4800]
              tunnel: w4791 -> [w4799]
              i -> [w4798]
              n3520 = Index Array(array=w4800, index (row)=w4798, index (col)=w4799) -> (element=w4797:string)
              n3521 = case shown="4" w4798 {
                tunnel: w4797 -> [w4801 w4802 _ w4803 w4804 w4805 w4806 w4807 w4808 w4809 w4810 w4811 w4812 w4813 w4814 w4815 w4816 w4817 w4818 w4819 w4820 w4821 w4822 w4823 w4824 w4825 w4826 w4827 w4828 _ _ w4829 w4830 w4831 w4832 w4833 w4834 w4843 w4850 w4857 w4864 w4868 w4871 w4874 w4876 w4878 w4879 w4880 w4881 w4882 w4883 w4884 w4885 w4886 w4887 w4888 w4889 w4890 w4891 w4892 w4893 w4894 w4895 w4896 w4897 w4898 w4899 w4900 w4901 w4902 w4903 w4904 w4905 w4906 w4907 w4908 w4909 w4910 w4911 w4912 w4913 w4914 w4915 w4916 w4917 w4918 w4919 w4920 w4921 w4922 w4923 w4924 w4925 w4926 w4927 w4928 w4929 w4930 w4931 w4932 w4933 w4934 w4935 w4936 w4937 _ w4938 w4939 w4940 w4941 w4942 w4943 w4944 w4945 w4946 w4947 w4948 w4949 w4950 _ w4951 w4952 w4953 w4954 w4955 w4956 _]
                frame 0 {
                  n3522 = local write "S"(w4801) -> ()
                }
                frame 1 {
                  n3523 = local write "S 2"(w4802) -> ()
                }
                frame 2 {
                }
                frame 3 {
                  n3524 = local write "S 4"(w4803) -> ()
                }
                frame 4 {
                  n3525 = property on="FILE" class="Str"("Caption.Text"=w4804) -> ()  [unwired: 2 in, 2 out]
                }
                frame 5 {
                  n3526 = property on="Fuel Discription :" class="Str"("Caption.Text"=w4805) -> ()  [unwired: 2 in, 2 out]
                }
                frame 6 {
                  n3527 = property on="Remarks :" class="Str"("Caption.Text"=w4806) -> ()  [unwired: 2 in, 2 out]
                }
                frame 7 {
                  n3528 = property on="Save & Continue" class="Bool (strict)"("Boolean Text.Text"=w4807) -> ()  [unwired: 2 in, 2 out]
                }
                frame 8 {
                }
                frame 9 {
                  n3529 = property on="Set Hz" class="DigNum (strict)"("Caption.Text"=w4809) -> ()  [unwired: 2 in, 2 out]
                }
                frame 10 {
                  "String 3" <- w4810
                }
                frame 11 {
                  n3530 = property on="NORMAL LOAD" class="DigNum (strict)"("Caption.Text"=w4811) -> ()  [unwired: 2 in, 2 out]
                }
                frame 12 {
                  "String 5" <- w4812
                }
                frame 13 {
                  n3531 = property on="Set Temp" class="DigNum (strict)"("Caption.Text"=w4813) -> ()  [unwired: 2 in, 2 out]
                }
                frame 14 {
                  n3532 = local write "S 15"(w4814) -> ()
                }
                frame 15 {
                  n3533 = property on="Set Rh" class="DigNum (strict)"("Caption.Text"=w4815) -> ()  [unwired: 2 in, 2 out]
                }
                frame 16 {
                  "String 13" <- w4816
                  "String 26" <- w4816
                }
                frame 17 {
                  n3534 = local write "S 18"(w4817) -> ()
                }
                frame 18 {
                  "String 17" <- w4818
                }
                frame 19 {
                  n3535 = property on="test time" class="DigNum (strict)"("Caption.Text"=w4819) -> ()  [unwired: 2 in, 2 out]
                }
                frame 20 {
                  "String 18" <- w4820
                  "String 22" <- w4820
                }
                frame 21 {
                  n3536 = property on="Elapsed time" class="DigNum (strict)"("Caption.Text"=w4821) -> ()  [unwired: 2 in, 2 out]
                }
                frame 22 {
                  n3537 = property on="Samplingtime 2" class="DigNum (strict)"("Caption.Text"=w4822) -> ()  [unwired: 2 in, 2 out]
                }
                frame 23 {
                  "String 21" <- w4823
                }
                frame 24 {
                  n3538 = property on="Countdown" class="DigNum (strict)"("Caption.Text"=w4824) -> ()  [unwired: 2 in, 2 out]
                }
                frame 25 {
                  n3539 = property on="Countdown 2" class="DigNum (strict)"("Caption.Text"=w4825) -> ()  [unwired: 2 in, 2 out]
                }
                frame 26 {
                  n3540 = property on="Engage" class="Bool (strict)"("Boolean Text.Text"=w4826) -> ()  [unwired: 2 in, 2 out]
                }
                frame 27 {
                  n3541 = property on="Boolean  4" class="Bool (strict)"("Boolean Text.Text"=w4827) -> ()  [unwired: 2 in, 2 out]
                }
                frame 28 {
                  n3542 = property on="Test \nStatus" class="Bool (strict)"("Boolean Text.Text"=w4828) -> ()  [unwired: 2 in, 2 out]
                }
                frame 29 {
                }
                frame 30 {
                }
                frame 31 {
                  n3543 = property on="FF Calibration g" class="WFGraph (strict)"("X Scale.Name Label.Text"=w4829) -> ()  [unwired: 2 in, 2 out]
                }
                frame 32 {
                  n3544 = property on="RSTCOF" class="Bool"("Boolean Text.Text"=w4830) -> ()  [unwired: 2 in, 2 out]
                  n3545 = property on="RST FF" class="Bool"("Boolean Text.Text"=w4830) -> ()  [unwired: 2 in, 2 out]
                  n3546 = property on="RST TEMP" class="Bool"("Boolean Text.Text"=w4830) -> ()  [unwired: 2 in, 2 out]
                  n3547 = property on="RSTV1 3" class="Bool"("Boolean Text.Text"=w4830) -> ()  [unwired: 2 in, 2 out]
                  n3548 = property on="rstv2" class="Bool"("Boolean Text.Text"=w4830) -> ()  [unwired: 2 in, 2 out]
                  n3549 = property on="RSTV1 2" class="Bool"("Boolean Text.Text"=w4830) -> ()  [unwired: 2 in, 2 out]
                  n3550 = property on="RST CP" class="Bool"("Boolean Text.Text"=w4830) -> ()  [unwired: 2 in, 2 out]
                }
                frame 33 {
                  "S 61" <- w4831
                }
                frame 34 {
                  "String 23" <- w4832
                }
                frame 35 {
                  n3551 = property on="Rh Before" class="DigNum (strict)"("Caption.Text"=w4833) -> ()  [unwired: 2 in, 2 out]
                }
                frame 36 {
                  n3552 = Match Pattern(string=w4834, regular expression=",") -> (before substring=→"bs":string, after substring=→"as":string)  [unwired: 1 in, 2 out]
                  n3553 = property on="Rh After" class="DigNum (strict)"("Caption.Text"=w4834) -> ()  [unwired: 2 in, 2 out]
                }
                frame 37 {
                  n3554 = Match Pattern(string=w4843, regular expression=",") -> (before substring=w4842:string, after substring=w4841:string)  [unwired: 1 in, 2 out]
                  "bs" <- w4842
                  "as" <- w4841
                  n3555 = Concatenate Strings(w4842, w4841) -> (w4838:string)
                  n3556 = property on="Humidity before test 2" class="DigNum (strict)"("Caption.Text"=w4838) -> ()  [unwired: 2 in, 2 out]
                  n3557 = property on="Humidity before test" class="DigNum (strict)"("Caption.Text"=w4838) -> ()  [unwired: 2 in, 2 out]
                  n3558 = Concatenate Strings(w4838, "=" ("string")) -> (w4839:string)
                  n3559 = local write "S 38"(w4839) -> ()
                }
                frame 38 {
                  n3560 = Match Pattern(string=w4850, regular expression=",") -> (before substring=w4849:string, after substring=w4848:string)  [unwired: 1 in, 2 out]
                  "bs" <- w4849
                  "as" <- w4848
                  n3561 = Concatenate Strings(w4849, w4848) -> (w4845:string)
                  n3562 = property on="Humidity after test 2" class="DigNum (strict)"("Caption.Text"=w4845) -> ()  [unwired: 2 in, 2 out]
                  n3563 = Concatenate Strings(w4845, "=" ("string")) -> (w4847:string)
                  n3564 = property on="Humidity after test" class="DigNum (strict)"("Caption.Text"=w4845) -> ()  [unwired: 2 in, 2 out]
                  n3565 = local write "S 39"(w4847) -> ()
                }
                frame 39 {
                  n3566 = Match Pattern(string=w4857, regular expression=",") -> (before substring=w4856:string, after substring=w4855:string)  [unwired: 1 in, 2 out]
                  "bs" <- w4856
                  "as" <- w4855
                  n3567 = Concatenate Strings(w4856, w4855) -> (w4852:string)
                  n3568 = property on="Temperature before test 2" class="DigNum (strict)"("Caption.Text"=w4852) -> ()  [unwired: 2 in, 2 out]
                  n3569 = property on="Temperature before test" class="DigNum (strict)"("Caption.Text"=w4852) -> ()  [unwired: 2 in, 2 out]
                  n3570 = Concatenate Strings(w4852, "=" ("string")) -> (→"String 34":string)
                }
                frame 40 {
                  n3571 = Match Pattern(string=w4864, regular expression=",") -> (before substring=w4863:string, after substring=w4862:string)  [unwired: 1 in, 2 out]
                  "bs" <- w4863
                  "as" <- w4862
                  n3572 = Concatenate Strings(w4863, w4862) -> (w4859:string)
                  n3573 = property on="Temperature after test 2" class="DigNum (strict)"("Caption.Text"=w4859) -> ()  [unwired: 2 in, 2 out]
                  n3574 = Concatenate Strings(w4859, "=" ("string")) -> (→"String 35":string)
                  n3575 = property on="Temperature after test" class="DigNum (strict)"("Caption.Text"=w4859) -> ()  [unwired: 2 in, 2 out]
                }
                frame 41 {
                  n3576 = property on="AVP" class="DigNum (strict)"("Caption.Text"=w4868) -> ()  [unwired: 2 in, 2 out]
                  n3577 = property on="AVP 2" class="DigNum (strict)"("Caption.Text"=w4868) -> ()  [unwired: 2 in, 2 out]
                  n3578 = Concatenate Strings(w4868, "=" ("string")) -> (→"String 36":string)
                }
                frame 42 {
                  n3579 = property on="MWSD" class="DigNum (strict)"("Caption.Text"=w4871) -> ()  [unwired: 2 in, 2 out]
                  n3580 = property on="MWSD 2" class="DigNum (strict)"("Caption.Text"=w4871) -> ()  [unwired: 2 in, 2 out]
                  n3581 = Concatenate Strings(w4871, "=" ("string")) -> (→"String 37":string)
                }
                frame 43 {
                  n3582 = property on="HCF 2" class="DigNum (strict)"("Caption.Text"=w4874) -> ()  [unwired: 2 in, 2 out]
                  n3583 = property on="HCF" class="DigNum (strict)"("Caption.Text"=w4874) -> ()  [unwired: 2 in, 2 out]
                  n3584 = Concatenate Strings(w4874, "=" ("string")) -> (→"String 38":string)
                }
                frame 44 {
                  n3585 = Concatenate Strings(w4876, "=" ("string")) -> (→"String 39":string)
                  n3586 = property on="WS1.4 2" class="DigNum (strict)"("Caption.Text"=w4876) -> ()  [unwired: 2 in, 2 out]
                  n3587 = property on="WS1.4" class="DigNum (strict)"("Caption.Text"=w4876) -> ()  [unwired: 2 in, 2 out]
                }
                frame 45 {
                  n3588 = property on="Save Results" class="Bool (strict)"("Boolean Text.Text"=w4878) -> ()  [unwired: 2 in, 2 out]
                }
                frame 46 {
                  n3589 = local write "S 47"(w4879) -> ()
                }
                frame 47 {
                  n3590 = local write "S 48"(w4880) -> ()
                }
                frame 48 {
                  n3591 = local write "S 49"(w4881) -> ()
                }
                frame 49 {
                  n3592 = local write "S 50"(w4882) -> ()
                }
                frame 50 {
                  n3593 = local write "S 51"(w4883) -> ()
                }
                frame 51 {
                  n3594 = local write "S 52"(w4884) -> ()
                }
                frame 52 {
                  n3595 = local write "S 53"(w4885) -> ()
                }
                frame 53 {
                  n3596 = local write "S 54"(w4886) -> ()
                }
                frame 54 {
                  n3597 = local write "S 55"(w4887) -> ()
                }
                frame 55 {
                  n3598 = local write "S 56"(w4888) -> ()
                }
                frame 56 {
                  n3599 = local write "S 57"(w4889) -> ()
                }
                frame 57 {
                  n3600 = local write "S 58"(w4890) -> ()
                }
                frame 58 {
                  n3601 = local write "S 59"(w4891) -> ()
                }
                frame 59 {
                  n3602 = local write "S 60"(w4892) -> ()
                }
                frame 60 {
                  n3603 = local write "S 62"(w4893) -> ()
                }
                frame 61 {
                  n3604 = local write "S 63"(w4894) -> ()
                }
                frame 62 {
                  n3605 = local write "S 64"(w4895) -> ()
                }
                frame 63 {
                  n3606 = local write "S 65"(w4896) -> ()
                }
                frame 64 {
                  n3607 = local write "S 66"(w4897) -> ()
                }
                frame 65 {
                  n3608 = local write "S 67"(w4898) -> ()
                }
                frame 66 {
                  n3609 = local write "S 68"(w4899) -> ()
                }
                frame 67 {
                  n3610 = local write "S 69"(w4900) -> ()
                }
                frame 68 {
                  n3611 = local write "S 70"(w4901) -> ()
                }
                frame 69 {
                  n3612 = local write "S 71"(w4902) -> ()
                }
                frame 70 {
                  n3613 = local write "S 72"(w4903) -> ()
                }
                frame 71 {
                  n3614 = local write "S 73"(w4904) -> ()
                }
                frame 72 {
                  n3615 = local write "S 74"(w4905) -> ()
                }
                frame 73 {
                  n3616 = local write "S 75"(w4906) -> ()
                }
                frame 74 {
                  n3617 = local write "S 76"(w4907) -> ()
                }
                frame 75 {
                  n3618 = local write "S 77"(w4908) -> ()
                }
                frame 76 {
                  n3619 = local write "S 78"(w4909) -> ()
                }
                frame 77 {
                  n3620 = local write "S 79"(w4910) -> ()
                }
                frame 79 {
                  n3621 = property on="Sample Temperature ( °C )" class="XYGraph (strict)"("Y Scale.Name Label.Text"=w4911) -> ()  [unwired: 2 in, 2 out]
                }
                frame 80 {
                  n3622 = local write "S 81"(w4912) -> ()
                  n3623 = property on="Humidity ( %RH )" class="XYGraph (strict)"("Y Scale.Name Label.Text"=w4912) -> ()  [unwired: 2 in, 2 out]
                }
                frame 78 {
                  n3624 = property on="Air Temperature  ( °C )" class="XYGraph (strict)"("X Scale.Name Label.Text"=w4913) -> ()  [unwired: 2 in, 2 out]
                  n3625 = property on="Humidity ( %RH )" class="XYGraph (strict)"("X Scale.Name Label.Text"=w4913) -> ()  [unwired: 2 in, 2 out]
                  n3626 = property on="Sample Temperature ( °C )" class="XYGraph (strict)"("X Scale.Name Label.Text"=w4913) -> ()  [unwired: 2 in, 2 out]
                  n3627 = property on="Coefficient Of Friction" class="XYGraph (strict)"("X Scale.Name Label.Text"=w4913) -> ()  [unwired: 2 in, 2 out]
                }
                frame 81 {
                  n3628 = property on="Air Temperature  ( °C )" class="XYGraph (strict)"("Y Scale.Name Label.Text"=w4914) -> ()  [unwired: 2 in, 2 out]
                }
                frame 82 {
                  n3629 = local write "S 84"(w4915) -> ()
                }
                frame 83 {
                  n3630 = local write "S 85"(w4916) -> ()
                }
                frame 84 {
                  n3631 = local write "S 86"(w4917) -> ()
                }
                frame 85 {
                  n3632 = local write "S 87"(w4918) -> ()
                }
                frame 86 {
                  n3633 = local write "S 88"(w4919) -> ()
                }
                frame 87 {
                  n3634 = property on="FF Calibration g" class="WFGraph (strict)"("Y Scale.Name Label.Text"=w4920) -> ()  [unwired: 2 in, 2 out]
                }
